vi "NISE.Set Device Property (U64).vi"(0 "SLSC Interface in":refnum<class "SLSC Interface.lvclass">, 5 "devices":refnum<k21>="$DefaultDevices", 7 "property":refnum<k21>, 9 "property value":u64, 11 "error in (no error)":errorcluster) -> (4 "SLSC Interface out":refnum<class "SLSC Interface.lvclass">, 15 "error out":errorcluster)   [LabVIEW 2016, in "SLSC Interface.lvclass"]
uses:
  SLSC Interface.lvclass
  NISE.Property Type.ctl
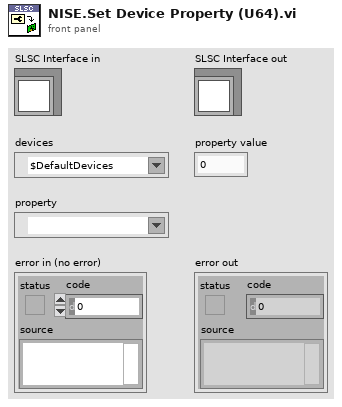
[diagram p1: front panel]
types:
  T1 = typedef "SLSC Interface.lvclass/NISE.Property Type.ctl" = enum16{"Bool", "DBL", "I32", "I64", "String", "U32", "U64", "1D Bool", "1D DBL", "1D I32", "1D I64", "1D String", "1D U32", "1D U64"}
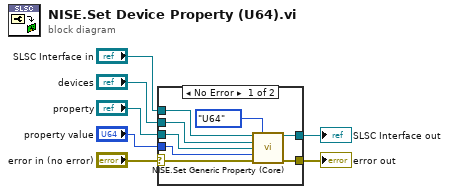
[diagram p0: block diagram]
diagram:
  n1 = case shown="No Error" "error in (no error)" {
    selector: "error in (no error)" -> [w11 w17]
    tunnel: [w12 w17] -> w6
    tunnel: [w14 w16] -> w4
    tunnel: "SLSC Interface in" -> [w15 w16]
    tunnel: "devices" -> [w9 _]
    tunnel: "property" -> [w10 _]
    tunnel: "property value" -> [w8 _]
    frame No Error {
      n2 = call "NISE.Set Generic Property (Core).vi"("SLSC Interface in"=w15, "property type"=NISE.Property_Type."U64", "resources"=w9, "property"=w10, "property value"=w8, "error in (no error)"=w11) -> ("SLSC Interface out"=w14:refnum<class "SLSC Interface.lvclass">, "error out"=w12:errorcluster)  [unwired: 8 in]
    }
    frame Error {
    }
  }
  "error out" <- w6
  "SLSC Interface out" <- w4
